vi "Управление звуком (SubVI).vi"(2 "Звук выстрела":bool, 3 "error in (no error)":errorcluster) -> (9 "error out":errorcluster)   [LabVIEW 2013]
doc: "Управление звуком при выстреле лазера"
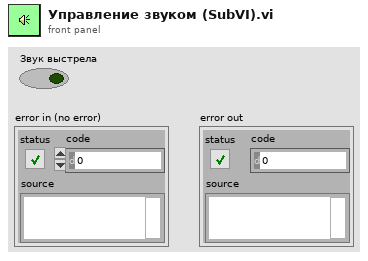
[diagram p1: front panel]
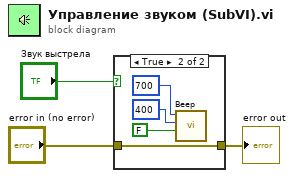
[diagram p0: block diagram]
diagram:
  n1 = case shown="True" "Звук выстрела" {
    tunnel: [w4 w5] -> w2
    tunnel: "error in (no error)" -> [w4 w5]
    frame False {
    }
    frame True {
      n2 = call <vilib>:"Beep.vi"("use system alert? (T)"=FALSE, "duration (msec)"=u32 400, "frequency (Hz)"=u32 700) -> ()  [unwired: 9 in]
    }
  }
  "error out" <- w2
